vi "Watchdog storage.vi"(7 "Command":T1, 10 "Watchdog Index":i32, 11 "Number of Watchdogs":i32) -> (1 "Skipped?":bool=TRUE, 2 "Max index":i32, 3 "Max Time":u32)   [LabVIEW 2014, in "RT Watchdog.lvlib"]
uses:
  RT Watchdog.lvlib
  Watchdog actions.ctl
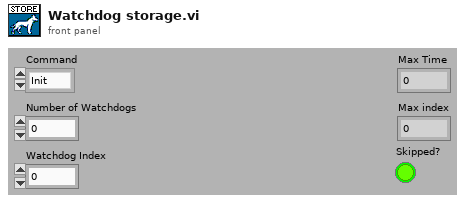
[diagram p1: front panel]
types:
  T1 = typedef "RT Watchdog.lvlib/Watchdog actions.ctl" = enum16{"Init", "Enable", "Service", "Disable", "Check"}
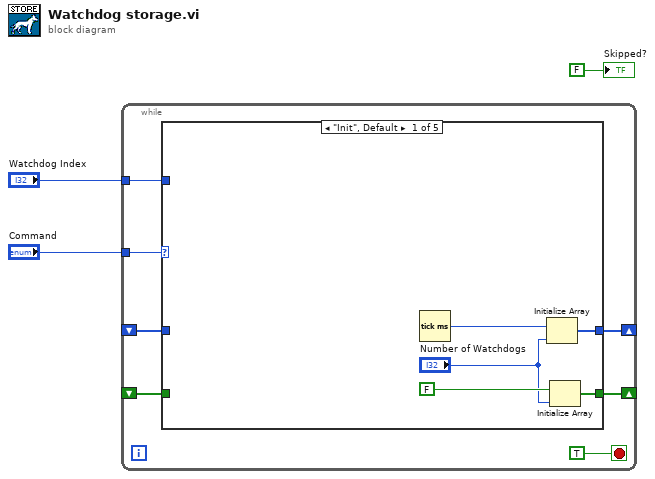
[diagram p0: block diagram]
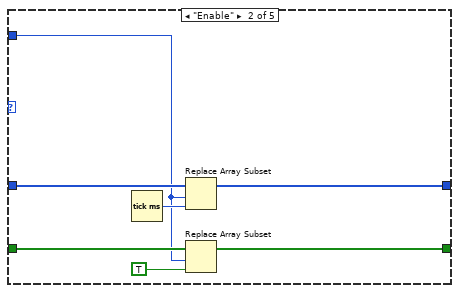
[diagram p2: hidden frame]
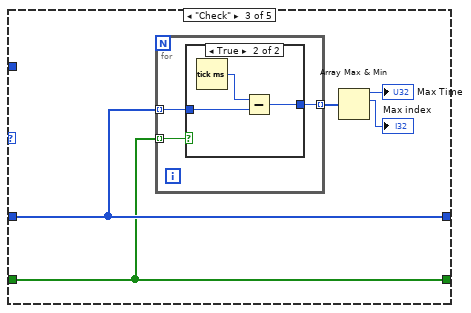
[diagram p3: hidden frame]
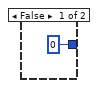
[diagram p4: hidden frame]
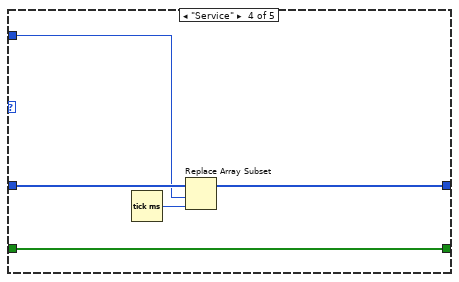
[diagram p5: hidden frame]
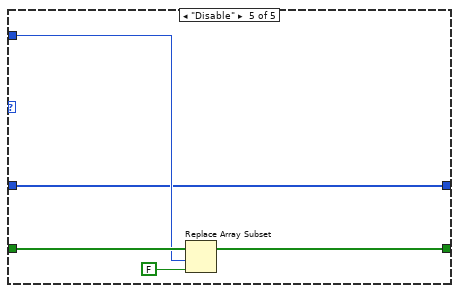
[diagram p6: hidden frame]
diagram:
  n1 = while {
    tunnel: "Command" -> [w10]
    shift-right: [w9] -> _
    shift-left: _ -> [w5]
    tunnel: "Watchdog Index" -> [w8]
    shift-right: [w7] -> _
    shift-left: _ -> [w6]
    stop <- TRUE stop-if-true
    n2 = case shown="\"Init\", Default" w10 {
      tunnel: [w11 w18 w27 w38 w40] -> w9
      tunnel: w8 -> [_ w16 _ w36 w42]
      tunnel: [w12 w20 w26 w35 w41] -> w7
      tunnel: w6 -> [_ w22 w26 w35 w44]
      tunnel: w5 -> [_ w19 w27 w39 w40]
      frame "Init", Default {
        n3 = Tick Count (ms)() -> (millisecond timer value=w15:u32)
        n4 = Initialize Array(w15, "Number of Watchdogs") -> (w11:u32[])
        n5 = Initialize Array(FALSE, "Number of Watchdogs") -> (w12:bool[])
      }
      frame "Enable" {
        n6 = Tick Count (ms)() -> (millisecond timer value=w17:u32)
        n7 = Replace Array Subset(array=w19, new element=w17, index=w16) -> (w18:u32[])
        n8 = Replace Array Subset(array=w22, new element=TRUE ("new element/subarray"), index=w16) -> (w20:bool[])
      }
      frame "Check" {
        n9 = for {
          tunnel: w27 -> [w29] mode=indexing
          tunnel: w26 -> [w30] mode=indexing
          tunnel: [w28] -> w25 mode=indexing
          n10 = case shown="True" w30 {
            tunnel: w29 -> [_ w34]
            tunnel: [u32 0 w32] -> w28
            frame False {
            }
            frame True {
              n11 = Tick Count (ms)() -> (millisecond timer value=w33:u32)
              n12 = Subtract(x=w33, y=w34) -> (x-y=w32:u32)
            }
          }
        }
        n13 = Array Max & Min(array=w25) -> (max value=→"Max Time":u32, max index (indices)=→"Max index":i32)  [unwired: 2 out]
      }
      frame "Service" {
        n14 = Tick Count (ms)() -> (millisecond timer value=w37:u32)
        n15 = Replace Array Subset(array=w39, new element=w37, index=w36) -> (w38:u32[])
      }
      frame "Disable" {
        n16 = Replace Array Subset(array=w44, new element=FALSE ("new element/subarray"), index=w42) -> (w41:bool[])
      }
    }
  }
  "Skipped?" <- FALSE ("Skipped?")
